vi "WriteDataToClass.vi"(8 "error in (no error)":errorcluster, 10 "Cluster":T1, 11 "DataClassNotifier out":refnum<notifier>) -> (0 "error out":errorcluster, 3 "DataClassNotifier out":refnum<notifier>)   [LabVIEW 2013, in "Data.lvclass"]
uses:
  Data.lvclass
  DataControlType.ctl
  DataVer1.lvclass/DataVer1.lvclass
  DataVer2.lvclass/DataVer2.lvclass
  DataVer3.lvclass/DataVer3.lvclass
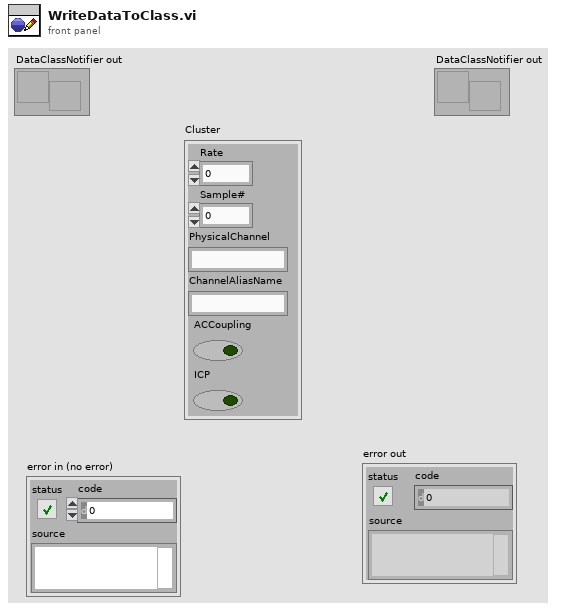
[diagram p1: front panel]
types:
  T1 = typedef "Data.lvclass/DataControlType.ctl" = cluster{"Rate":dbl, "Sample#":dbl, "PhysicalChannel":string, "ChannelAliasName":string, "ACCoupling":bool, "ICP":bool}
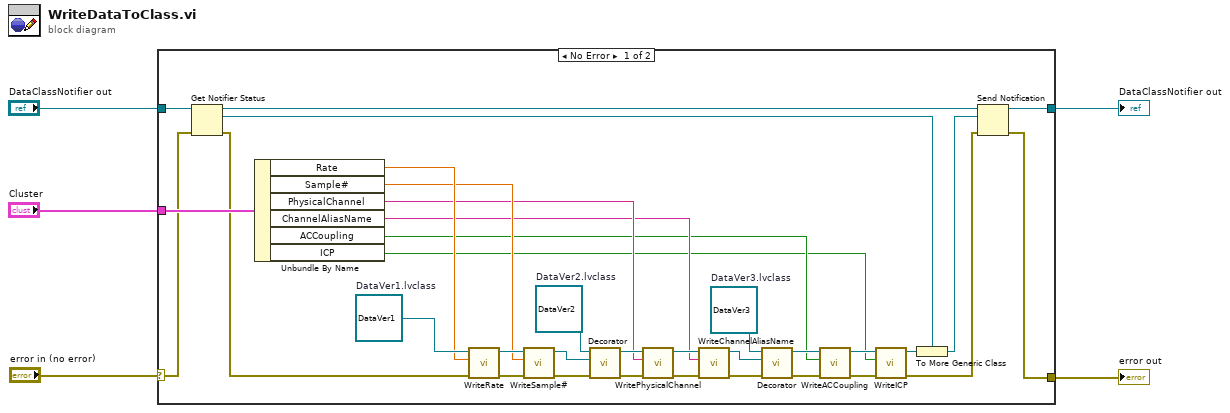
[diagram p0: block diagram]
diagram:
  n1 = case shown="No Error" "error in (no error)" {
    selector: "error in (no error)" -> [w7 w41]
    tunnel: "Cluster" -> [w29 _]
    tunnel: [w15 w40] -> w3
    tunnel: "DataClassNotifier out" -> [w10 w40]
    tunnel: [w14 w41] -> w1
    frame No Error {
      w39 = refnum<class "DataVer3.lvclass"> refnum  # DataVer3.lvclass
      w33 = refnum<class "DataVer2.lvclass"> refnum  # DataVer2.lvclass
      w38 = refnum<class "DataVer1.lvclass"> refnum  # DataVer1.lvclass
      n2 = Get Notifier Status(notifier=w10, error in (no error)=w7) -> (notifier out=w9:refnum<notifier>, current notification=w8:refnum<class "Data.lvclass">, error out=w6:errorcluster)  [unwired: 2 out]
      n3 = Unbundle By Name(w29) -> ("Rate"=w28:dbl, "Sample#"=w27:dbl, "PhysicalChannel"=w26:string, "ChannelAliasName"=w25:string, "ACCoupling"=w24:bool, "ICP"=w23:bool)
      n4 = call-dynamic "WriteRate.vi"("error in (no error)"=w6, "Rate"=w28, "DataVer1 in"=w38) -> ("error out"=w22:errorcluster, "DataVer1 out"=w37:refnum<class "DataVer1.lvclass">)  [unwired: 7 in]
      n5 = call-dynamic "WriteSample#.vi"("error in (no error)"=w22, "Sample#"=w27, "DataVer1 in"=w37) -> ("error out"=w21:errorcluster, "DataVer1 out"=w35:refnum<class "DataVer1.lvclass">)  [unwired: 7 in]
      n6 = call-dynamic "Decorator.vi"("error in (no error)"=w21, "DecoratorData in"=w35, "DataVer2 in"=w33) -> ("error out"=w20:errorcluster, "DataVer2 out"=w34:refnum<class "DataVer2.lvclass">)  [unwired: 7 in]
      n7 = call-dynamic "WritePhysicalChannel.vi"("error in (no error)"=w20, "PhysicalChannel"=w26, "DataVer2 in"=w34) -> ("error out"=w19:errorcluster, "DataVer2 out"=w36:refnum<class "DataVer2.lvclass">)  [unwired: 7 in]
      n8 = call-dynamic "WriteChannelAliasName.vi"("error in (no error)"=w19, "ChannelAliasName"=w25, "DataVer2 in"=w36) -> ("error out"=w18:errorcluster, "DataVer2 out"=w32:refnum<class "DataVer2.lvclass">)  [unwired: 7 in]
      n9 = call-dynamic "Decorator.vi"("error in (no error)"=w18, "DecoratorData in"=w32, "DataVer3 in"=w39) -> ("error out"=w17:errorcluster, "DataVer3 out"=w31:refnum<class "DataVer3.lvclass">)  [unwired: 7 in]
      n10 = call-dynamic "WriteACCoupling.vi"("error in (no error)"=w17, "ACCoupling"=w24, "DataVer3 in"=w31) -> ("error out"=w16:errorcluster, "DataVer3 out"=w30:refnum<class "DataVer3.lvclass">)  [unwired: 7 in]
      n11 = call-dynamic "WriteICP.vi"("error in (no error)"=w16, "ICP"=w23, "DataVer3 in"=w30) -> ("error out"=w12:errorcluster, "DataVer3 out"=w13:refnum<class "DataVer3.lvclass">)  [unwired: 7 in]
      n12 = To More Generic Class(target class=w8, reference=w13) -> (generic class reference=w11:refnum<class "Data.lvclass">)
      n13 = Send Notification(notification=w11, notifier=w9, error in (no error)=w12) -> (notifier out=w15:refnum<notifier>, error out=w14:errorcluster)
    }
    frame Error {
    }
  }
  "error out" <- w1
  "DataClassNotifier out" <- w3
